vi "Calculate Range Array.vi"(11 "2D Array In":dbl[][](array[numeric])) -> (1 "Ranges":dbl[](array[numeric]), 2 "Average Range":dbl, 3 "2D array Out":dbl[][](array[numeric]))   [LabVIEW 2018, in "GRR Core.lvclass"]
uses:
  GRR Core.lvclass
  <vilib>/Analysis/baseanly.llb/Mean (DBL).vi
  <vilib>/Analysis/NI_AALBase.lvlib
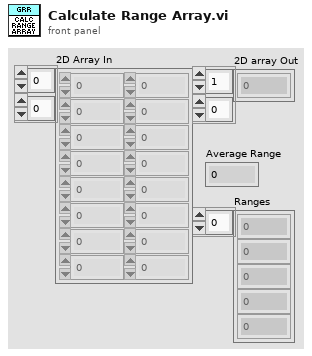
[diagram p1: front panel]
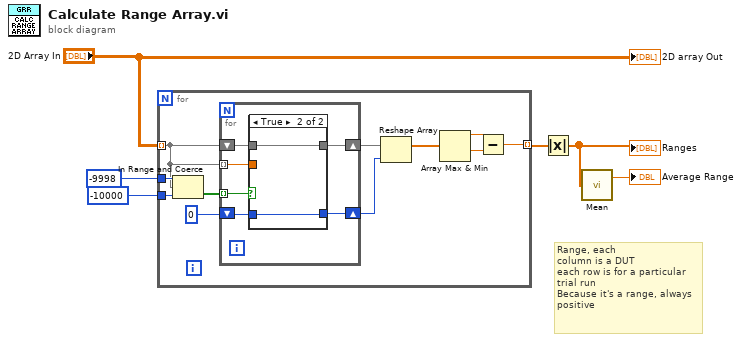
[diagram p0: block diagram]
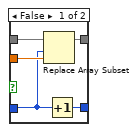
[diagram p2: hidden frame]
diagram:
  # "Range, each\ncolumn is a DUT\neach row is for a particular \ntrial run\nBecause it's a range, always\npositive"
  n1 = for {
    tunnel: "2D Array In" -> [w11] mode=indexing
    tunnel: [w15] -> w6 mode=indexing
    tunnel: -9998 -> [w14]
    tunnel: -10000 -> [w13]
    n2 = In Range and Coerce(upper limit=w14, x=w11, lower limit=w13) -> (In Range?=w12:bool[])  [unwired: 1 out]
    n3 = for {
      shift-right: [w23] -> w9
      shift-left: w11 -> [w22]
      tunnel: w12 -> [w21] mode=indexing
      tunnel: w11 -> [w20] mode=indexing
      shift-right: [w18] -> w7
      shift-left: 0 -> [w19]
      n4 = case shown="True" w21 {
        tunnel: [w28 w29] -> w23
        tunnel: w22 -> [w27 w29]
        tunnel: w20 -> [w26 _]
        tunnel: w19 -> [w25 w30]
        tunnel: [w24 w30] -> w18
        frame False {
          n5 = Replace Array Subset(array=w27, new element=w26, index=w25) -> (w28:dbl[])
          n6 = Increment(x=w25) -> (x+1=w24:i32)
        }
        frame True {
        }
      }
    }
    n7 = Reshape Array(w9, w7) -> (w8:dbl[])
    n8 = Array Max & Min(array=w8) -> (max value=w17:dbl, min value=w16:dbl)  [unwired: 2 out]
    n9 = Subtract(x=w17, y=w16) -> (x-y=w15:dbl)
  }
  n10 = Absolute Value(x=w6) -> (abs(x)=w5:dbl[])
  "Ranges" <- w5
  n11 = call-poly <vilib>:"Mean.vi"("X"=w5) -> ("mean"=→"Average Range":dbl)  [unwired: 1 out]
  "2D array Out" <- "2D Array In"
